vi "Get To Mul.vi"(8 "error in (no error)":errorcluster, 11 "ByRef Mul in":refnum<class "ByRef Mul.lvclass">) -> (0 "error out":errorcluster, 2 "To Mul":dbl, 3 "ByRef Mul out":refnum<class "ByRef Mul.lvclass">)   [LabVIEW 2012, in "ByRef Mul.lvclass"]
uses:
  ByRef Mul.lvclass
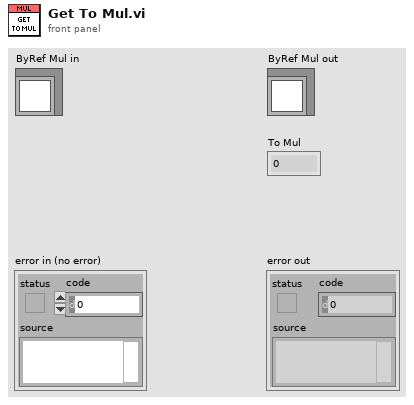
[diagram p1: front panel]
types:
  T1 = typedef "ByRef Mul.lvclass/Ref Data.ctl" = cluster{"To Mul":dbl}
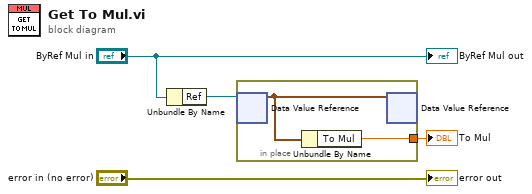
[diagram p0: block diagram]
diagram:
  n1 = Unbundle By Name("ByRef Mul in") -> ("Ref"=w3:refnum<data-value>)
  n2 = in-place {
    in-place-border: [w5] -> w1
    n3 = in-place-dvr #1(w3) -> (w6:T1)  [unwired: 1 out]
    n4 = Unbundle By Name(w6) -> ("To Mul"=w5:dbl)
    n5 = in-place-dvr #1(w6) -> ()  [unwired: 2 out]
  }
  "To Mul" <- w1
  "error out" <- "error in (no error)"
  "ByRef Mul out" <- "ByRef Mul in"
